vi "Phasics intensity array to image.vi"(7 "Intensity in":sgl[][](array[numeric]), 8 "error in (no error)":errorcluster, 11 "Phasics Camera in":refnum<class "Phasics Camera.lvclass">) -> (0 "error out":errorcluster, 3 "Phasics Camera out":refnum<class "Phasics Camera.lvclass">)   [LabVIEW 2013, in "Phasics Camera.lvclass"]
uses:
  Phasics Camera.lvclass
  Phasics Camera.lvclass/Phasics Camera.ctl
  CompressAndUpdate(IMAQ Image).vi
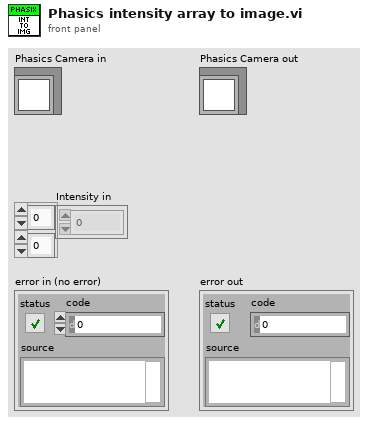
[diagram p1: front panel]
types:
  T1 = typedef "IMAQ Image.ctl" = refnum<image>
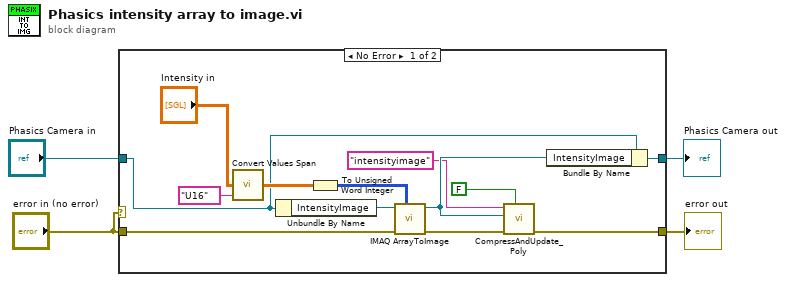
[diagram p0: block diagram]
diagram:
  n1 = case shown="No Error" "error in (no error)" {
    tunnel: "error in (no error)" -> [w14 w19]
    tunnel: [w9 w19] -> w4
    tunnel: "Phasics Camera in" -> [w7 w18]
    tunnel: [w5 w18] -> w2
    frame No Error {
      n2 = call "Convert Values Span.vi"("Input Array"="Intensity in", "Data type"="U16") -> ("Output Array"=w10:sgl[][])  [unwired: 5 in]
      n3 = Unbundle By Name(w7) -> ("IntensityImage"=w6:T1)
      n4 = To Unsigned Word Integer(number=w10) -> (unsigned 16bit integer=w16:u16[][])
      n5 = call "IMAQ ArrayToImage"("Image Pixels (U16)"=w16, "error in (no error)"=w14, "Image"=w6) -> ("error out"=w15:errorcluster, "Image Out"=w17:T1)  [unwired: 7 in]
      n6 = call-poly "CompressAndUpdate_Poly.vi"("force CVT update (false)"=FALSE, "error in"=w15, "IMAQ Image"=w17, "command or variable name"="intensityimage") -> ("error out"=w9:errorcluster)  [unwired: 7 in]
      n7 = Bundle By Name(cluster=w7, "IntensityImage"=w17) -> (w5:refnum<class "Phasics Camera.lvclass">)
    }
    frame Error {
    }
  }
  "error out" <- w4
  "Phasics Camera out" <- w2
